vi "ConsoleView.vi"(10 "Return Queue":refnum<queue>, 11 "ConsoleView Sink in":refnum<class "ConsoleView.lvclass">) -> ()   [LabVIEW 2018, in "MVA Framework.lvlib" / "ConsoleView.lvlib" / "ConsoleView.lvclass"]
uses:
  ConsoleView.lvclass
  Composed Log/Types/MessageCluster.ctl
  Composed Log/Composed Log.lvlib
  Composed Log/Types/Log Level.ctl
  Composed Log/Types/Log Packet.ctl
  TypeDef/FilterConfig.ctl
  TypeDef/String Config.ctl
panel:
  out "View":string
  in  "Defer Shutdown?":bool
  in  "Filters Enabled?":bool
  in  "Filter":bool
  in  "Autoscroll?":bool=TRUE
  in  "Items to Show":i32=1024
  in  "Clear":bool
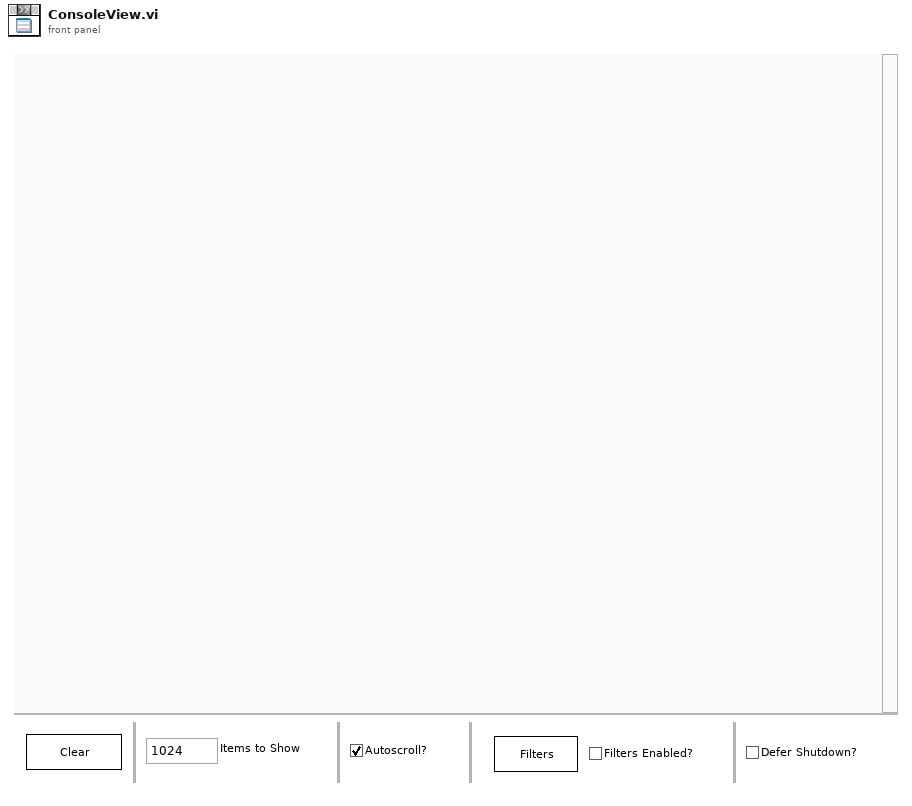
[diagram p1: front panel]
types:
  T1 = enum32{"Invalid", "Standard", "Closed", "Hidden", "Minimized", "Maximized"}
  T2 = typedef "MVA Framework.lvlib/ConsoleView.lvlib/ConsoleView.lvclass/String Config.ctl" = cluster{"BG Color":u32, "Text Color":u32, "Font Size":u32, "Bold?":bool}
  T3 = typedef "MVA Framework.lvlib/ConsoleView.lvlib/ConsoleView.lvclass/FilterConfig.ctl" = cluster{"Level Filter":cluster{"Warning":bool, "Debug":bool, "Info":bool, "Error":bool, "Critical":bool}, "Source Filter":cluster{"Source":string, "Exclude Match?":bool, "Exact Match?":bool}, "Keyword Filter":cluster{"Keywords":string[], "Exclude Match?":bool}}
  T4 = typedef "MVA Framework.lvlib/Composed Log.lvlib/Log Packet.ctl" = cluster{"Data To Log":string, "Source":string, "Event Level":T5, "Event Time":timestamp}
  T5 = typedef "MVA Framework.lvlib/Composed Log.lvlib/Log Level.ctl" = enum16{"Debug", "Info", "Warning", "Error", "Critical"}
  T6 = typedef "MVA Framework.lvlib/Composed Log.lvlib/MessageCluster.ctl" = cluster{"Message":string, "Data":variant}
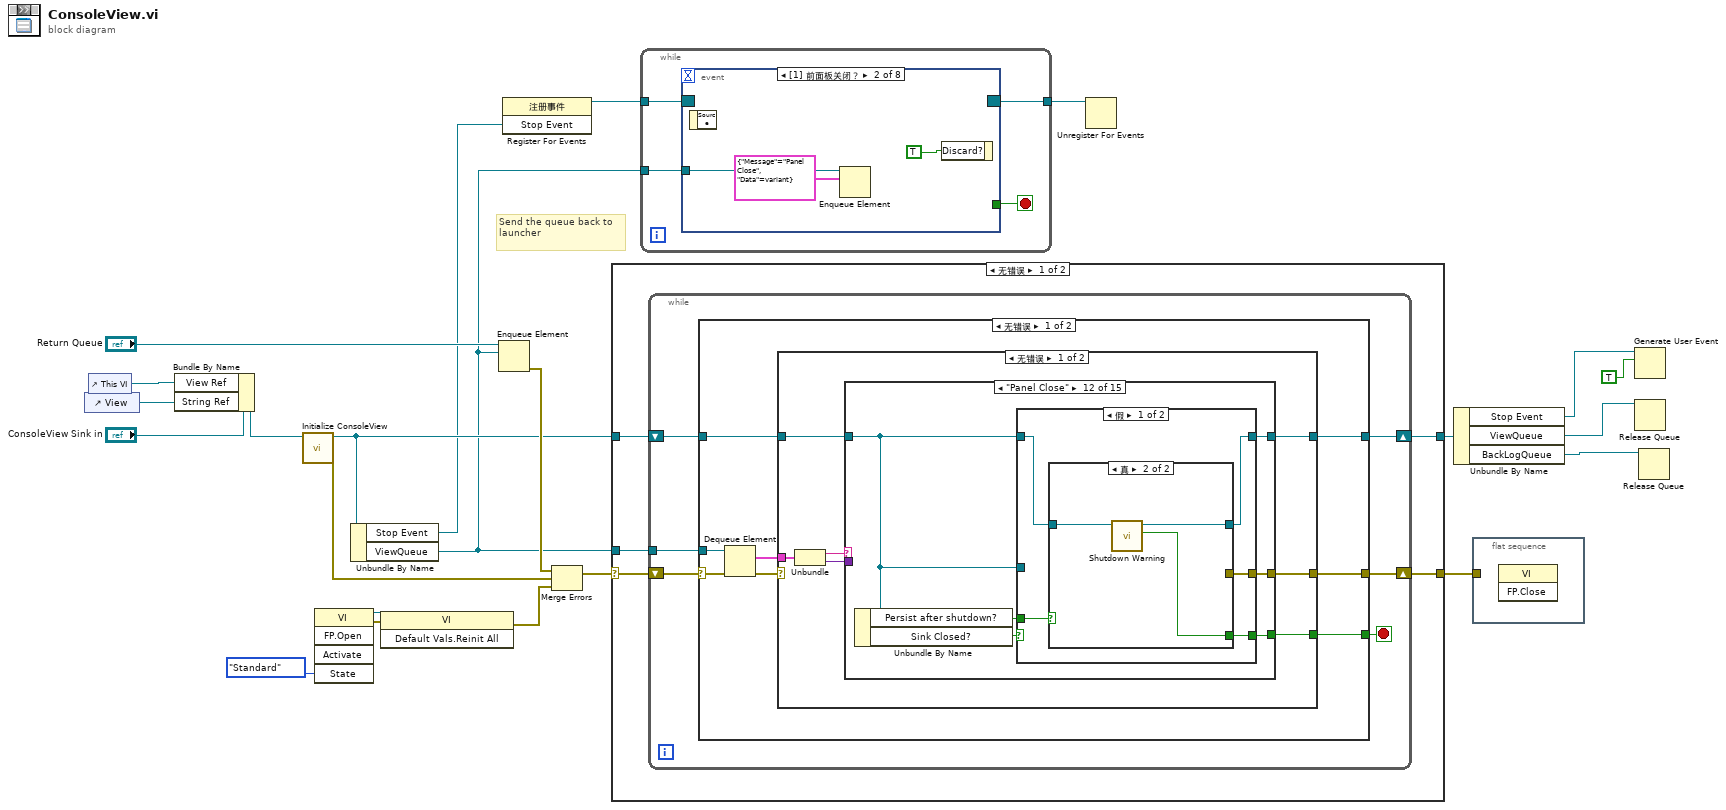
[diagram p0: block diagram]
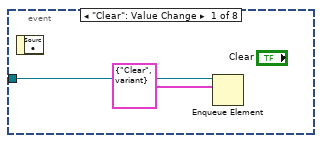
[diagram p2: hidden frame]
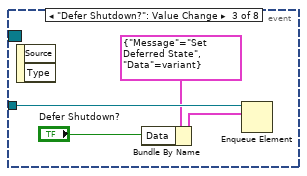
[diagram p3: hidden frame]
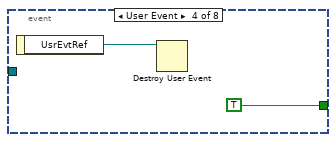
[diagram p4: hidden frame]
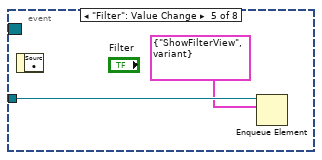
[diagram p5: hidden frame]
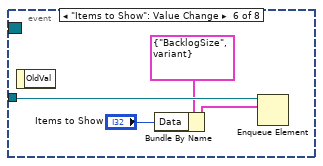
[diagram p6: hidden frame]
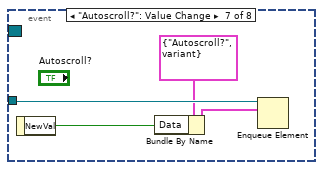
[diagram p7: hidden frame]
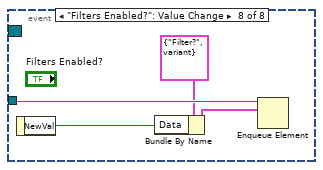
[diagram p8: hidden frame]
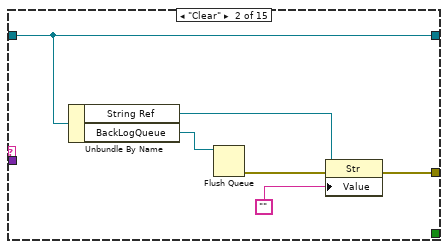
[diagram p10: hidden frame]
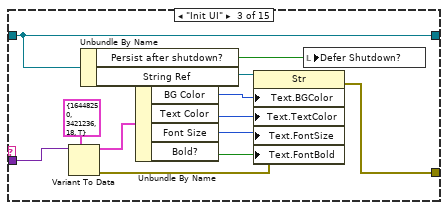
[diagram p11: hidden frame]
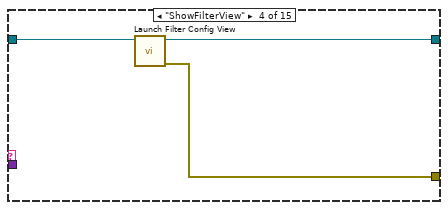
[diagram p12: hidden frame]
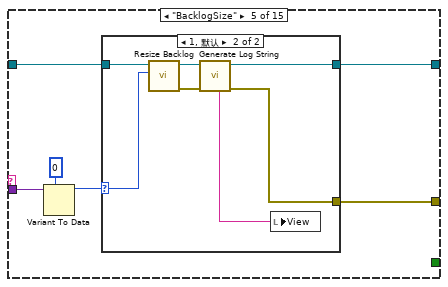
[diagram p13: hidden frame]
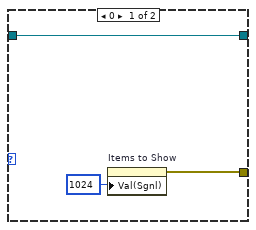
[diagram p14: hidden frame]
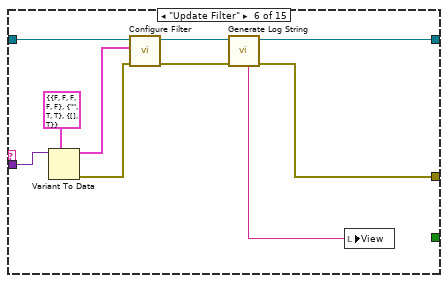
[diagram p15: hidden frame]
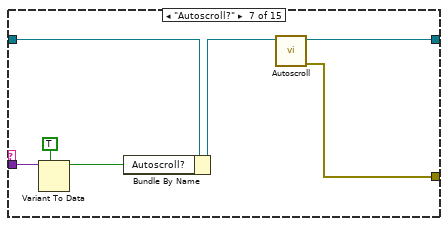
[diagram p16: hidden frame]
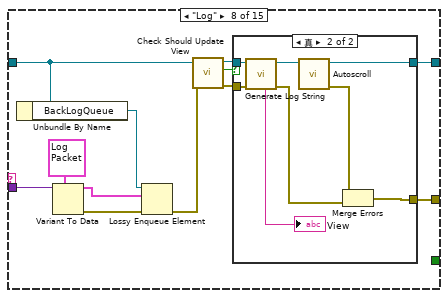
[diagram p17: hidden frame]
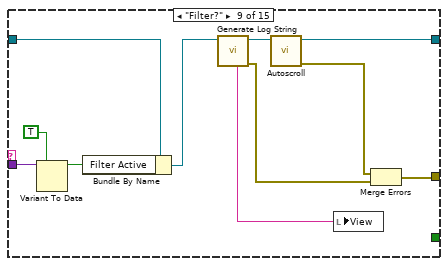
[diagram p19: hidden frame]
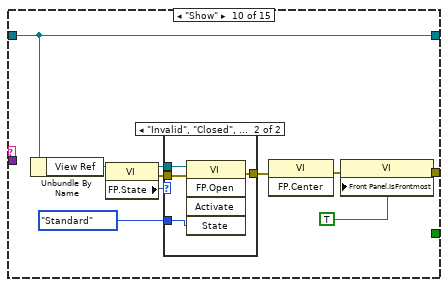
[diagram p20: hidden frame]
diagram:
  # "Send the queue back to launcher"
  n1 = control-ref of="View"() -> (w13:refnum<vi>)
  n2 = control-ref of="This VI"() -> (w8:refnum<vi>)
  n3 = Bundle By Name(cluster="ConsoleView Sink in", "View Ref"=w8, "String Ref"=w13) -> (w12:refnum<class "ConsoleView.lvclass">)
  n4 = call "Initialize ConsoleView.vi"("ConsoleView in"=w12) -> ("error out"=w10:errorcluster, "ConsoleView out"=w11:refnum<class "ConsoleView.lvclass">)  [unwired: 9 in]
  n5 = invoke class="VI" method="FP.Open"("State"=T1."Standard") -> (reference out=w15:refnum<vi>, error out=w14:errorcluster)  [unwired: 4 in, 3 out]
  n6 = Unbundle By Name(w11) -> ("Stop Event"=w3:refnum<user-event>, "ViewQueue"=w4:refnum<queue>)
  n7 = invoke class="VI" method="Default Vals.Reinit All"(reference=w15, error in=w14) -> (error out=w9:errorcluster)  [unwired: 1 in, 2 out]
  n8 = Enqueue Element(queue="Return Queue", element=w4) -> (error out=w22:errorcluster)  [unwired: 2 in, 2 out]
  n9 = register-events(w3) -> (reference out=w18:refnum<event-registration>)  [unwired: 2 in, 1 out]
  n10 = Merge Errors(w22, w10, w9) -> (w21:errorcluster)
  n11 = case shown="无错误" w21 {
    selector: w21 -> [w28 w193]
    tunnel: w4 -> [w25 _]
    tunnel: w11 -> [w27 w192]
    tunnel: [w26 w193] -> w17
    tunnel: [w24 w192] -> w7
    frame No Error {
      n12 = while {
        tunnel: w25 -> [w34]
        shift-right: [w31] -> w26
        shift-left: w28 -> [w32]
        shift-right: [w29] -> w24
        shift-left: w27 -> [w30]
        stop <- w33 stop-if-true
        n13 = case shown="无错误" w32 {
          selector: w32 -> [w39 w191]
          tunnel: w34 -> [w35 _]
          tunnel: [w40 TRUE] -> w33
          tunnel: [w38 w191] -> w31
          tunnel: w30 -> [w37 w189]
          tunnel: [w36 w189] -> w29
          frame No Error {
            n14 = Dequeue Element(queue=w35, error in (no error)=w39) -> (element=w42:T6, error out=w41:errorcluster)  [unwired: 1 in, 2 out]
            n15 = case shown="无错误" w41 {
              selector: w41 -> [_ w188]
              tunnel: w42 -> [w49 _]
              tunnel: [w46 _] -> w40
              tunnel: [w43 w188] -> w38
              tunnel: w37 -> [w45 w187]
              tunnel: [w44 w187] -> w36
              frame No Error {
                n16 = Unbundle(w49) -> ("Message"=w48:string, "Data"=w47:variant)
                n17 = case shown="\"Panel Close\"" w48 {
                  tunnel: w47 -> [_ _ w66 _ w76 w97 w101 w116 w137 _ _ _ w178 _ _]
                  tunnel: [_ _ _ _ _ _ _ _ _ _ _ w157 _ TRUE w182] -> w46
                  tunnel: w45 -> [w50 w52 w68 w71 w77 w95 w104 w109 w134 w145 w154 w160 w179 w180 w184]
                  tunnel: [w50 w52 w68 w70 w73 w91 w103 w115 w131 w145 w154 w159 w176 w180 w186] -> w44
                  tunnel: [_ w55 w63 w69 w72 w89 w98 w114 w128 w139 w155 w161 _ _ _] -> w43
                  frame "False", Default {
                  }
                  frame "Clear" {
                    n18 = Unbundle By Name(w52) -> ("String Ref"=w51:refnum<vi>, "BackLogQueue"=w54:refnum<queue>)
                    n19 = Flush Queue(queue=w54) -> (error out=w53:errorcluster)  [unwired: 1 in, 2 out]
                    n20 = property class="Str"(reference=w51, error in=w53, "Value"="") -> (error out=w55:errorcluster)  [unwired: 1 out]
                  }
                  frame "Init UI" {
                    n21 = Variant To Data(type=T2 {"BG Color"=16448250, "Text Color"=3421236, "Font Size"=18, "Bold?"=TRUE} ("UI Config"), Variant=w66) -> (data=w62:T2, error out=w64:errorcluster)  [unwired: 1 in]
                    n22 = Unbundle By Name(w68) -> ("Persist after shutdown?"=w57:bool, "String Ref"=w67:refnum<vi>)
                    n23 = Unbundle By Name(w62) -> ("BG Color"=w61:u32, "Text Color"=w60:u32, "Font Size"=w59:u32, "Bold?"=w58:bool)
                    n24 = property class="Str"(reference=w67, error in=w64, "Text.BGColor"=w61, "Text.TextColor"=w60, "Text.FontSize"=w59, "Text.FontBold"=w58) -> (error out=w63:errorcluster)  [unwired: 1 out]
                    n25 = local write "Defer Shutdown?"(w57) -> ()
                  }
                  frame "ShowFilterView" {
                    n26 = call "Launch Filter Config View.vi"("ConsoleView in"=w71) -> ("error out"=w69:errorcluster, "ConsoleView out"=w70:refnum<class "ConsoleView.lvclass">)  [unwired: 9 in]
                  }
                  frame "BacklogSize" {
                    n27 = Variant To Data(type=0 ("Backlog Size"), Variant=w76) -> (data=w74:i32)  [unwired: 1 in, 1 out]
                    n28 = case shown="1, 默认" w74 {
                      selector: w74 -> [_ w86]
                      tunnel: w77 -> [w80 w87]
                      tunnel: [w80 w82] -> w73
                      tunnel: [w79 w84] -> w72
                      frame 0 {
                        n29 = property on="Items to Show" class="DigNum (严格)"("Val(Sgnl)"=1024 ("Items to Show")) -> (error out=w79:errorcluster)  [unwired: 2 in, 1 out]
                      }
                      frame 1, Default {
                        n30 = call "Resize Backlog.vi"("Backlog Size"=w86, "ConsoleView Sink in"=w87) -> ("error out"=w85:errorcluster, "ConsoleView Sink out"=w83:refnum<class "ConsoleView.lvclass">)  [unwired: 8 in]
                        n31 = call "Generate Log String.vi"("error in (no error)"=w85, "ConsoleView Sink in"=w83) -> ("error out"=w84:errorcluster, "ConsoleView Sink out"=w82:refnum<class "ConsoleView.lvclass">, "Log String"=w81:string)  [unwired: 7 in]
                        n32 = local write "View"(w81) -> ()
                      }
                    }
                  }
                  frame "Update Filter" {
                    n33 = Variant To Data(type=T3 {"Level Filter"={"Warning"=FALSE, "Debug"=FALSE, "Info"=FALSE, "Error"=FALSE, "Critical"=FALSE}, "Source Filter"={"Source"="", "Exclude Match?"=TRUE, "Exact Match?"=TRUE}, "Keyword Filter"={"Keywords"=[], "Exclude Match?"=TRUE}} ("Current Filter Settings"), Variant=w97) -> (data=w94:T3, error out=w93:errorcluster)  [unwired: 1 in]
                    n34 = call "Configure Filter.vi"("error in (no error)"=w93, "Current Filter Settings"=w94, "ConsoleView Sink in"=w95) -> ("error out"=w90:errorcluster, "ConsoleView Sink out"=w92:refnum<class "ConsoleView.lvclass">)  [unwired: 7 in]
                    n35 = call "Generate Log String.vi"("error in (no error)"=w90, "ConsoleView Sink in"=w92) -> ("error out"=w89:errorcluster, "ConsoleView Sink out"=w91:refnum<class "ConsoleView.lvclass">, "Log String"=w88:string)  [unwired: 7 in]
                    n36 = local write "View"(w88) -> ()
                  }
                  frame "Autoscroll?" {
                    n37 = Variant To Data(type=TRUE, Variant=w101) -> (data=w99:bool)  [unwired: 1 in, 1 out]
                    n38 = Bundle By Name(cluster=w104, "Autoscroll?"=w99) -> (w102:refnum<class "ConsoleView.lvclass">)
                    n39 = call "Autoscroll.vi"("ConsoleView Sink in"=w102) -> ("error out"=w98:errorcluster, "ConsoleView Sink out"=w103:refnum<class "ConsoleView.lvclass">)  [unwired: 9 in]
                  }
                  frame "Log" {
                    n40 = Unbundle By Name(w109) -> ("BackLogQueue"=w113:refnum<queue>)
                    n41 = Variant To Data(type=T4 {"Data To Log"="", "Source"="", "Event Level"=enum."Debug", "Event Time"=timestamp(0 s since 1904-01-01)} ("element"), Variant=w116) -> (data=w111:T4, error out=w110:errorcluster)  [unwired: 1 in]
                    n42 = Lossy Enqueue Element(queue=w113, element=w111, error in (no error)=w110) -> (error out=w108:errorcluster)  [unwired: 3 out]
                    n43 = call "Check Should Update View.vi"("error in (no error)"=w108, "ConsoleView in"=w109) -> ("error out"=w107:errorcluster, "Log?"=w105:bool, "ConsoleView out"=w106:refnum<class "ConsoleView.lvclass">)  [unwired: 7 in]
                    n44 = case shown="真" w105 {
                      tunnel: [w118 w126] -> w115
                      tunnel: [w117 w124] -> w114
                      tunnel: w106 -> [w118 w120]
                      tunnel: w107 -> [w117 w119]
                      frame False {
                      }
                      frame True {
                        n45 = call "Generate Log String.vi"("error in (no error)"=w119, "ConsoleView Sink in"=w120) -> ("error out"=w122:errorcluster, "ConsoleView Sink out"=w123:refnum<class "ConsoleView.lvclass">, "Log String"=→"View":string)  [unwired: 7 in]
                        n46 = call "Autoscroll.vi"("ConsoleView Sink in"=w123) -> ("error out"=w125:errorcluster, "ConsoleView Sink out"=w126:refnum<class "ConsoleView.lvclass">)  [unwired: 9 in]
                        n47 = Merge Errors(w125, w122) -> (w124:errorcluster)
                      }
                    }
                  }
                  frame "Filter?" {
                    n48 = Variant To Data(type=TRUE, Variant=w137) -> (data=w135:bool)  [unwired: 1 in, 1 out]
                    n49 = Bundle By Name(cluster=w134, "Filter Active"=w135) -> (w133:refnum<class "ConsoleView.lvclass">)
                    n50 = call "Generate Log String.vi"("ConsoleView Sink in"=w133) -> ("error out"=w129:errorcluster, "ConsoleView Sink out"=w132:refnum<class "ConsoleView.lvclass">, "Log String"=w127:string)  [unwired: 8 in]
                    n51 = call "Autoscroll.vi"("ConsoleView Sink in"=w132) -> ("error out"=w130:errorcluster, "ConsoleView Sink out"=w131:refnum<class "ConsoleView.lvclass">)  [unwired: 9 in]
                    n52 = local write "View"(w127) -> ()
                    n53 = Merge Errors(w130, w129) -> (w128:errorcluster)
                  }
                  frame "Show" {
                    n54 = Unbundle By Name(w145) -> ("View Ref"=w144:refnum<vi>)
                    n55 = property class="VI"(reference=w144) -> (reference out=w143:refnum<vi>, error out=w141:errorcluster, "FP.State"=w142:T1)  [unwired: 1 in]
                    n56 = case shown="\"Invalid\", \"Closed\", \"Hidden\"" w142 {
                      tunnel: T1."Standard" ("State") -> [_ w152]
                      tunnel: [w148 w151] -> w146
                      tunnel: w143 -> [_ w150]
                      tunnel: w141 -> [w148 w149]
                      frame "Standard", Default {
                      }
                      frame "Invalid", "Closed", "Hidden" {
                        n57 = invoke class="VI" method="FP.Open"(reference=w150, error in=w149, "State"=w152) -> (error out=w151:errorcluster)  [unwired: 2 in, 4 out]
                      }
                    }
                    n58 = invoke class="VI" method="FP.Center"(error in=w146) -> (error out=w140:errorcluster)  [unwired: 2 in, 2 out]
                    n59 = property class="VI"(error in=w140, "Front Panel.IsFrontmost"=TRUE ("Front Panel Window:Is Frontmost")) -> (error out=w139:errorcluster)  [unwired: 1 in, 1 out]
                  }
                  frame "Hide" {
                    n60 = Unbundle By Name(w154) -> ("View Ref"=w153:refnum<vi>)
                    n61 = invoke class="VI" method="FP.Close"(reference=w153) -> (error out=w155:errorcluster)  [unwired: 2 in, 2 out]
                  }
                  frame "Panel Close" {
                    n62 = Unbundle By Name(w160) -> ("Persist after shutdown?"=w156:bool, "Sink Closed?"=w158:bool)
                    n63 = case shown="假" w158 {
                      selector: w158 -> [_ w173]
                      tunnel: [w166 _] -> w161
                      tunnel: w160 -> [_ _]
                      tunnel: w160 -> [w164 w174]
                      tunnel: [w163 w174] -> w159
                      tunnel: [w162 w173] -> w157
                      tunnel: w156 -> [w165 _]
                      frame False {
                        n64 = case shown="真" w165 {
                          tunnel: [w169 _] -> w166
                          tunnel: w164 -> [w167 w172]
                          tunnel: [w167 w171] -> w163
                          tunnel: [_ w170] -> w162
                          frame False {
                            n65 = Unbundle By Name(w167) -> ("View Ref"=w168:refnum<vi>)
                            n66 = invoke class="VI" method="FP.Close"(reference=w168) -> (error out=w169:errorcluster)  [unwired: 2 in, 2 out]
                          }
                          frame True {
                            n67 = call "Shutdown Warning.vi"("ConsoleView Sink in"=w172) -> ("Shutdown?"=w170:bool, "ConsoleView Sink Out"=w171:refnum<class "ConsoleView.lvclass">)  [unwired: 9 in]
                          }
                        }
                      }
                      frame True {
                      }
                    }
                  }
                  frame "Set Deferred State" {
                    n68 = Variant To Data(type=TRUE, Variant=w178) -> (data=w175:bool)  [unwired: 1 in, 1 out]
                    n69 = Bundle By Name(cluster=w179, "Persist after shutdown?"=w175) -> (w176:refnum<class "ConsoleView.lvclass">)
                  }
                  frame "Stop" {
                  }
                  frame "Sink Closed" {
                    n70 = Unbundle By Name(w184) -> ("Persist after shutdown?"=w183:bool)
                    n71 = Bundle By Name(cluster=w184, "Sink Closed?"=TRUE) -> (w186:refnum<class "ConsoleView.lvclass">)
                    n72 = Not(x=w183) -> (.not. x?=w182:bool)
                  }
                }
              }
              frame Error {
              }
            }
          }
          frame Error {
          }
        }
      }
    }
    frame Error {
    }
  }
  n73 = while {
    tunnel: w4 -> [w197]
    tunnel: w18 -> [w195]
    tunnel: [w194] -> w16
    stop <- w196 stop-if-true
    n74 = event shown="[1] 前面板关闭？" {
      selector: w195 -> [_ _ _ _ _ _ _ _]
      dyn-events: [_ _ _ _ _ _ _ _] -> w194
      timeout: _ -> [_ _ _ _ _ _ _ _]
      tunnel: w197 -> [w199 w201 w206 _ w210 w214 w218 w222]
      tunnel: [_ _ _ TRUE ("Discard?") _ _ _ _] -> w196
      event "Clear": Value Change {
        n75 = event-data() -> ()  [unwired: 1 in, 1 out]
        n76 = Enqueue Element(queue=w199, element=T6 {"Message"="Clear", "Data"=variant}) -> ()  [unwired: 2 in, 3 out]
      }
      event Panel Close? {
        n77 = event-data() -> ()  [unwired: 1 in, 1 out]
        n78 = Enqueue Element(queue=w201, element=T6 {"Message"="Panel Close", "Data"=variant}) -> ()  [unwired: 2 in, 3 out]
        n79 = event-data("Discard?"=TRUE) -> ()  [unwired: 1 in, 1 out]
      }
      event "Defer Shutdown?": Value Change {
        n80 = event-data() -> ()  [unwired: 1 in, 2 out]
        n81 = Bundle By Name(cluster=T6 {"Message"="Set Deferred State", "Data"=variant} ("element"), "Data"="Defer Shutdown?") -> (w204:T6)
        n82 = Enqueue Element(queue=w206, element=w204) -> ()  [unwired: 2 in, 3 out]
      }
      event User Event {
        n83 = event-data() -> ("UsrEvtRef"=w207:refnum<user-event>)  [unwired: 1 in]
        n84 = Destroy User Event(user event=w207) -> ()  [unwired: 1 in, 1 out]
      }
      event "Filter": Value Change {
        n85 = event-data() -> ()  [unwired: 1 in, 1 out]
        n86 = Enqueue Element(queue=w210, element=T6 {"Message"="ShowFilterView", "Data"=variant}) -> ()  [unwired: 2 in, 3 out]
      }
      event "Items to Show": Value Change {
        n87 = event-data() -> ()  [unwired: 1 in, 1 out]
        n88 = Bundle By Name(cluster=T6 {"Message"="BacklogSize", "Data"=variant} ("element"), "Data"="Items to Show") -> (w212:T6)
        n89 = Enqueue Element(queue=w214, element=w212) -> ()  [unwired: 2 in, 3 out]
      }
      event "Autoscroll?": Value Change {
        n90 = event-data() -> ("NewVal"=w215:bool)  [unwired: 1 in]
        n91 = Bundle By Name(cluster=T6 {"Message"="Autoscroll?", "Data"=variant} ("element"), "Data"=w215) -> (w216:T6)
        n92 = Enqueue Element(queue=w218, element=w216) -> ()  [unwired: 2 in, 3 out]
      }
      event "Filters Enabled?": Value Change {
        n93 = event-data() -> ("NewVal"=w219:bool)  [unwired: 1 in]
        n94 = Bundle By Name(cluster=T6 {"Message"="Filter?", "Data"=variant} ("element"), "Data"=w219) -> (w220:T6)
        n95 = Enqueue Element(queue=w222, element=w220) -> ()  [unwired: 2 in, 3 out]
      }
    }
  }
  n96 = Unregister For Events(event registration refnum=w16) -> ()  [unwired: 1 in, 1 out]
  n97 = Unbundle By Name(w7) -> ("Stop Event"=w1:refnum<user-event>, "ViewQueue"=w5:refnum<queue>, "BackLogQueue"=w6:refnum<queue>)
  n98 = flat-sequence {
    tunnel: w17 -> [_]
    frame #0 {
      n99 = invoke class="VI" method="FP.Close"() -> ()  [unwired: 3 in, 3 out]
    }
  }
  n100 = Generate User Event(user event=w1, event data cluster=TRUE ("event data")) -> ()  [unwired: 2 in, 2 out]
  n101 = Release Queue(queue=w5) -> ()  [unwired: 2 in, 3 out]
  n102 = Release Queue(queue=w6) -> ()  [unwired: 2 in, 3 out]
